vi "Load LayerStitch.vi"(3 "errorIN":errorcluster) -> (0 "error OUT":errorcluster, 2 "stitchType":string[](array[string]))   [LabVIEW 2010]
uses:
  BIMS_Collector Globals.vi
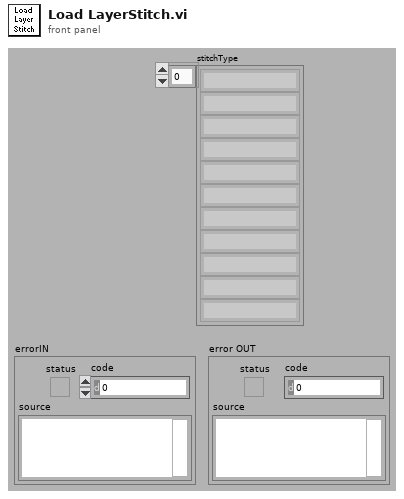
[diagram p1: front panel]
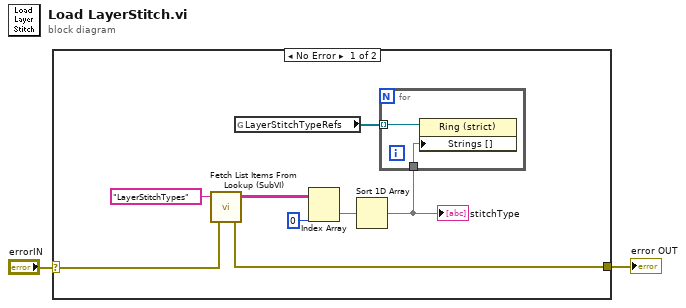
[diagram p0: block diagram]
diagram:
  n1 = case shown="No Error" "errorIN" {
    selector: "errorIN" -> [w6 w13]
    tunnel: [w5 w13] -> w2
    frame No Error {
      n2 = call "Fetch List Items From Lookup (SubVI).vi"("error IN"=w6, "Query"="LayerStitchTypes" ("lookup table name")) -> ("error OUT"=w5:errorcluster, "recordset data"=w10:string[][])  [unwired: 2 out]
      n3 = global read "BIMS_Collector Globals.vi" "LayerStitchTypeRefs"() -> (w3:refnum<vi>[])
      n4 = Index Array(array=w10, index (col)=0 ("disabled index (col)")) -> (element=w8:string[])  [unwired: 1 in]
      n5 = Sort 1D Array(array=w8) -> (sorted array=w7:string[])
      "stitchType" <- w7
      n6 = for {
        tunnel: w3 -> [w12] mode=indexing
        tunnel: w7 -> [w11]
        n7 = property class="Ring (strict)"(reference=w12, "Strings []"=w11) -> ()  [unwired: 1 in, 2 out]
      }
    }
    frame Error {
    }
  }
  "error OUT" <- w2
